vi "Sea-Level SWI Read Bit.vi"(6 "Access Mode (Relative)":T1, 7 "Adapter Info":T2, 8 "error in (no error)":errorcluster, 10 "Bit Number":u32, 11 "Handle":i32) -> (0 "error out":errorcluster, 2 "State":bool, 3 "Handle Out":i32, 4 "Error Code":T3)   [LabVIEW 2011]
uses:
  TypeDefs/Sea-Level SWI Error Code.ctl
  TypeDefs/Sea-Level SWI Adapter Info.ctl
  TypeDefs/Sea-Level SWI Access Mode.ctl
  SeaIo32.dll
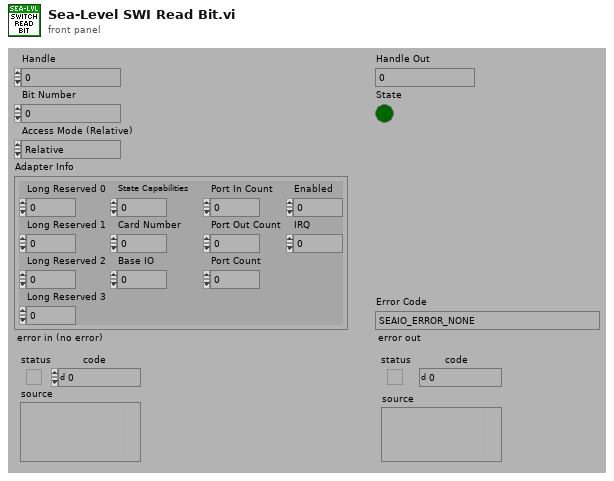
[diagram p1: front panel]
types:
  T1 = typedef "Sea-Level SWI Access Mode.ctl" = enum16{"Relative", "Absolute"}
  T2 = typedef "Sea-Level SWI Adapter Info.ctl" = cluster{"Long Reserved 0":i32, "Long Reserved 1":i32, "Long Reserved 2":i32, "Long Reserved 3":i32, "State Capabilities":i32, "Card Number":i16, "Base IO":i16, "Port In Count":i8, "Port Out Count":i8, "Port Count":i8, "Enabled":i8, "IRQ":i16}
  T3 = typedef "Sea-Level SWI Error Code.ctl" = enum16{"SEAIO_ERROR_NONE", "SEAIO_ERROR_PARAM", "SEAIO_ERROR_NOT_SUPPORTED", "SEAIO_ERROR_PORT_NOT_OPEN", "SEAIO_ERROR_INVALID_NAME", "SEAIO_ERROR_SHARING_VIOLATION", "SEAIO_ERROR_DRIVER_TYPE", "SEAIO_ERROR_BUFFER", "SEAIO_ERROR_INCOMPLETE", "SEAIO_ERROR_GENERAL", "SEAIO_ERROR_IO_PENDING", "SEAIO_ERROR_NO_TXBUFFER", "SEAIO_ERROR_INVALID_DEVICE_REQUEST", "SEAIO_ERROR_INVALID_HANDLE", "SEAIO_ERROR_CANCELED", "SEAIO_ERROR_LAST", "SEAIO_ERROR_NO_MEMORY", "SEAIO_ERROR_BUSY"}
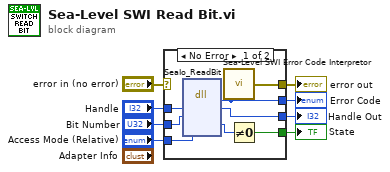
[diagram p0: block diagram]
diagram:
  n1 = case shown="No Error" "error in (no error)" {
    selector: "error in (no error)" -> [_ w17]
    tunnel: [w16 _] -> w8
    tunnel: [w15 w17] -> w7
    tunnel: "Handle" -> [w14 _]
    tunnel: [w13 _] -> w4
    tunnel: "Bit Number" -> [w12 _]
    tunnel: [w10 _] -> w2
    tunnel: "Access Mode (Relative)" -> [w9 _]
    frame No Error {
      n2 = dll-call lib="C:/Development/Spartan/www/drivers/SWI/Sea-Level/SeaIo32.dll" fn="SeaIo_ReadBit"("Handle"=w14, "Bit Number"=w12, "Access Mode"=w9) -> ("Error Code"=w16:i32, "Handle"=w13:i32, "State"=w11:i16)  [unwired: 4 in, 4 out]
      n3 = call "Sea-Level SWI Error Code Interpretor.vi"("Error Code"=w16) -> ("error out"=w15:errorcluster)
      n4 = Not Equal To 0?(x=w11) -> (x != 0?=w10:bool)
    }
    frame Error {
    }
  }
  "Error Code" <- w8
  "error out" <- w7
  "Handle Out" <- w4
  "State" <- w2
